vi "Read All.vi"(6 "Per Read Size":u64=1024 max=30000, 8 "Error In":errorcluster, 10 "Max Read Size":u64=1024, 11 "SFTP File In":refnum<class "SFTP File.lvclass">) -> (0 "Error Out":errorcluster, 2 "Data":u8[](array[numeric]), 3 "SFTP File Out":refnum<class "SFTP File.lvclass">)   [LabVIEW 2018, in "Toolkit.lvlib" / "SFTP File.lvclass"]
doc: "Reads binary data from a SFTP file represented by this SFTP File object in chunks, or blocks, until the total read size is reached. This VI should be used if the <B>Total Read Size</B> is greater than 30KB because of a hard-coded per-read maximum of 30KB set in the libssh2 shared library."
uses:
  SFTP File.lvclass
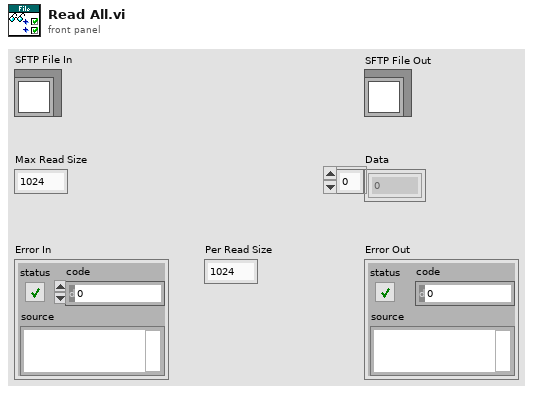
[diagram p1: front panel]
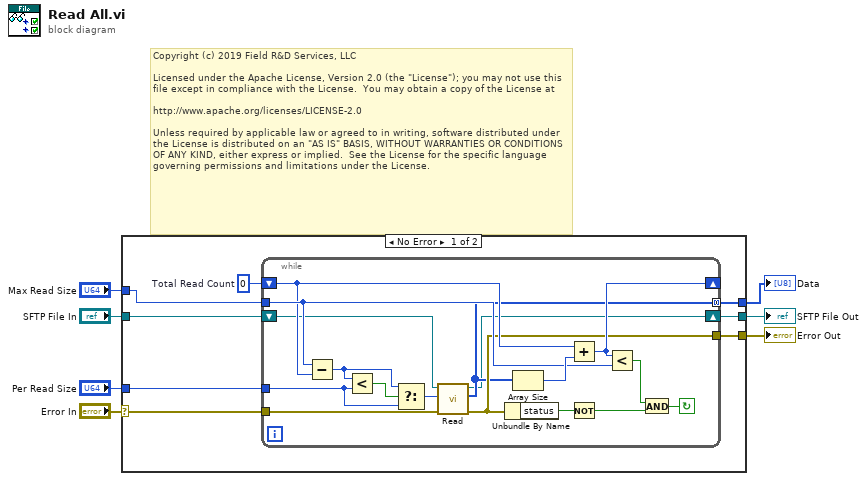
[diagram p0: block diagram]
diagram:
  # "Copyright (c) 2019 Field R&D Services, LLC\n\nLicensed under the Apache License, Version 2.0 (the \"License\"); you may not use this file except in compliance with the License.  You may obtain a copy of the License at\n\nhttp://www.apache.org/licenses/LICENSE-2.0\n\nUnless required by applicable law or agreed to in writing, software distributed under the License is distributed on an \"AS IS\" BASIS, WITHOUT WARRANTIES OR CONDITIONS OF ANY KIND, either express or implied.  See the License for the specific language governing permissions and limitations under the License."
  n1 = case shown="No Error" "Error In" {
    selector: "Error In" -> [w11 w34]
    tunnel: "Max Read Size" -> [w14 _]
    tunnel: "Per Read Size" -> [w13 _]
    tunnel: [w12 _] -> w5
    tunnel: [w10 w34] -> w4
    tunnel: "SFTP File In" -> [w9 w33]
    tunnel: [w8 w33] -> w1
    frame No Error {
      w15 = u64 0  # Total Read Count
      n2 = while {
        shift-right: [w16] -> w8
        shift-left: w9 -> [w17]
        tunnel: [w18] -> w12 mode=concatenating
        shift-right: [w31] -> _
        shift-left: w15 -> [w29]
        tunnel: w14 -> [w30]
        tunnel: w13 -> [w26]
        tunnel: w11 -> [w21]
        tunnel: [w20] -> w10
        stop <- w22 continue-if-true
        n3 = Subtract(x=w30, y=w29) -> (x-y=w27:u64)
        n4 = Less?(x=w27, y=w26) -> (x < y?=w28:bool)
        n5 = Select(t=w27, s=w28, f=w26) -> (s? t:f=w19:u64)
        n6 = call "Read.vi"("Error In"=w21, "Max Data Length"=w19, "SFTP File In"=w17) -> ("Error Out"=w20:errorcluster, "Data"=w18:u8[], "SFTP File Out"=w16:refnum<class "SFTP File.lvclass">)  [unwired: 6 in]
        n7 = Unbundle By Name(w20) -> ("status"=w25:bool)
        n8 = Array Size(array=w18) -> (size(s)=w32:i32)
        n9 = Add(x=w29, y=w32) -> (x+y=w31:u64)
        n10 = Not(x=w25) -> (.not. x?=w23:bool)
        n11 = Less?(x=w31, y=w30) -> (x < y?=w24:bool)
        n12 = And(x=w24, y=w23) -> (x .and. y?=w22:bool)
      }
    }
    frame Error {
    }
  }
  "Data" <- w5
  "Error Out" <- w4
  "SFTP File Out" <- w1
